vi "white_p.vi"(11 "Array":u8[](array[numeric])) -> (0 "White":bool)   [LabVIEW 2013]
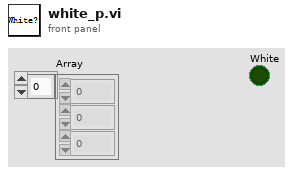
[diagram p1: front panel]
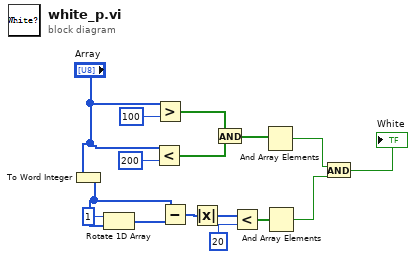
[diagram p0: block diagram]
diagram:
  n1 = To Word Integer(number="Array") -> (16bit integer=w8:i16[])
  n2 = Rotate 1D Array(1:w8, 2:1 ("n")) -> (0:w10:i16[])
  n3 = Less?(x="Array", y=u8 200) -> (x < y?=w13:bool[])
  n4 = Greater?(x="Array", y=u8 100) -> (0:w14:bool[])
  n5 = Subtract(x=w8, y=w10) -> (x-y=w7:i16[])
  n6 = Absolute Value(x=w7) -> (abs(x)=w6:i16[])
  n7 = And(x=w14, y=w13) -> (x .and. y?=w12:bool[])
  n8 = Less?(x=w6, y=i16 20) -> (x < y?=w3:bool[])
  n9 = And Array Elements(Boolean array=w12) -> (logical AND=w4:bool)
  n10 = And Array Elements(Boolean array=w3) -> (logical AND=w1:bool)
  n11 = And(x=w4, y=w1) -> (x .and. y?=→"White":bool)
